vi "G-DataType-To-Go.vi"(8 "error in (no error)":errorcluster, 11 "CMD":variant) -> (0 "error out":errorcluster, 3 "result string":string)   [LabVIEW 2020, in "Generate-Go-CMD.lvlib"]
uses:
  Generate-Go-CMD.lvlib
  <vilib>/Utility/Data Type/NI_Data Type.lvlib
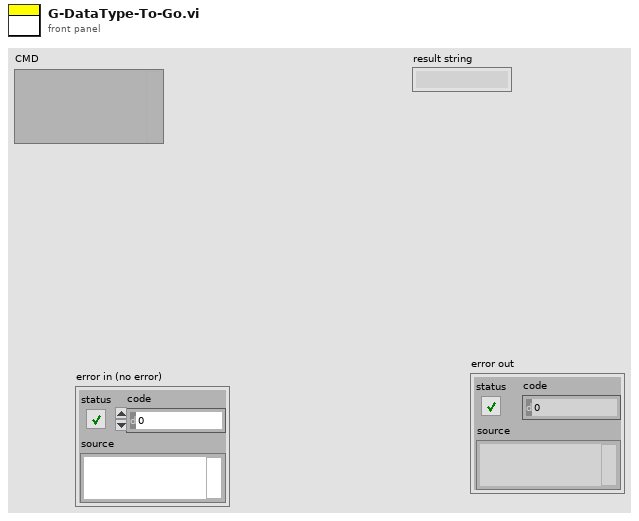
[diagram p1: front panel]
types:
  T1 = typedef "NI_Data Type.lvlib/Data Type.ctl" = enum8{"Invalid Type", "Void", "I8", "I16", "I32", "I64", "U8", "U16", "U32", "U64", "Single Float", "Double Float", "Extended Float", "Single Complex", "Double Complex", "Extended Complex", "Enum U8", "Enum U16", "Enum U32", "Enum U64", "Single Float With Unit", "Double Float With Unit", "Extended Float With Unit", "Single Complex with Unit", "Double Complex with Unit", "Extended Complex with Unit", "Boolean", "String", "Path", "Picture", "Tag", "Array", "Cluster", "Variant", "LV Variant", "Waveform", "Timestamp", "Digital Waveform", "Digital Data", "ExpressData", "Refnum", "External Data", "VI", "Poly VI", "LabVIEW Class Instance", "Fixed Point", "Set Collection", "Map Collection"}
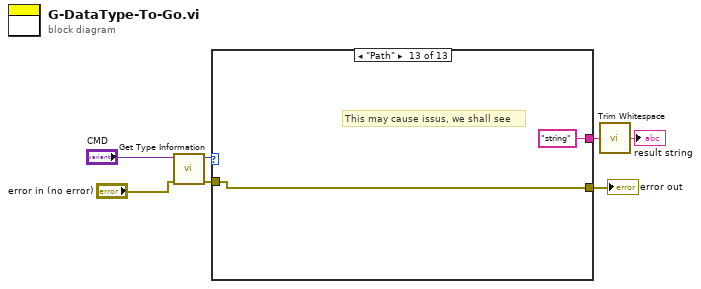
[diagram p0: block diagram]
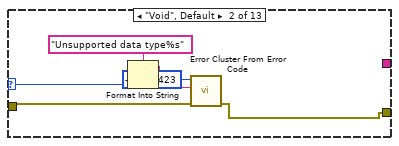
[diagram p3: hidden frame]
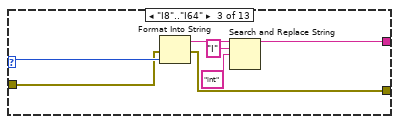
[diagram p4: hidden frame]
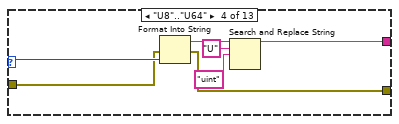
[diagram p5: hidden frame]
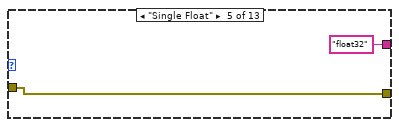
[diagram p6: hidden frame]
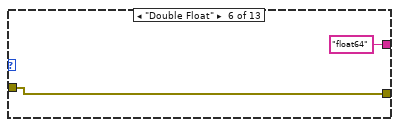
[diagram p7: hidden frame]
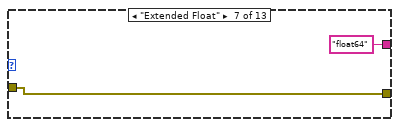
[diagram p8: hidden frame]
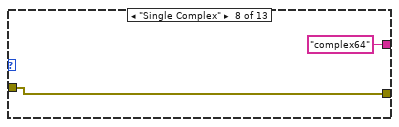
[diagram p9: hidden frame]
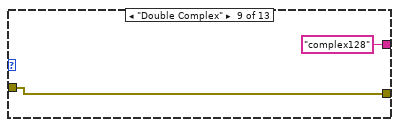
[diagram p10: hidden frame]
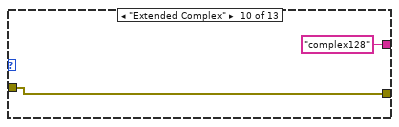
[diagram p11: hidden frame]
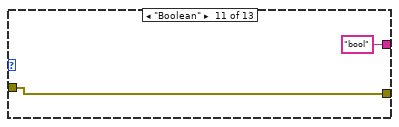
[diagram p12: hidden frame]
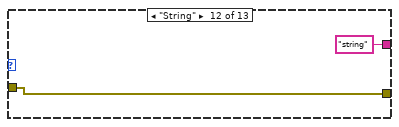
[diagram p13: hidden frame]
diagram:
  n1 = call <vilib>:"Get Type Information.vi"("error in (no error)"="error in (no error)", "variant"="CMD") -> ("error out"=w3:errorcluster, "type"=w5:T1)  [unwired: 5 in, 3 out]
  n2 = case shown="\"Path\"" w5 {
    selector: w5 -> [_ w13 w21 w28 _ _ _ _ _ _ _ _ _]
    tunnel: [_ _ w17 w24 "float32" ("result string") "float64" ("result string") "float64" ("result string") "complex64" ("result string") "complex128" ("result string") "complex128" ("result string") "bool" ("result string") "string" ("result string") "string" ("result string")] -> w4
    tunnel: w3 -> [w8 w14 w16 w23 w29 w31 w33 w35 w37 w39 w41 w43 w45]
    tunnel: [w8 w10 w15 w22 w29 w31 w33 w35 w37 w39 w41 w43 w45] -> w2
    frame "Invalid Type" {
    }
    frame "Void", Default {
      n3 = Format Into String(format string="Unsupported data type%s", w13) -> (resulting string=w12:string)  [unwired: 2 in, 1 out]
      n4 = call <vilib>:"Error Cluster From Error Code.vi"("error in (no error)"=w14, "error message (\"\")"=w12, "error code (0)"=-98328423) -> ("error out"=w10:errorcluster)  [unwired: 6 in]
    }
    frame "I8".."I64" {
      n5 = Format Into String(error in=w16, w21) -> (resulting string=w20:string, error out=w15:errorcluster)  [unwired: 2 in]
      n6 = Search and Replace String(input string=w20, search string="I", replace string="int" ("search string")) -> (result string=w17:string)  [unwired: 5 in, 3 out]
    }
    frame "U8".."U64" {
      n7 = Format Into String(error in=w23, w28) -> (resulting string=w27:string, error out=w22:errorcluster)  [unwired: 2 in]
      n8 = Search and Replace String(input string=w27, search string="U", replace string="uint" ("search string")) -> (result string=w24:string)  [unwired: 5 in, 3 out]
    }
    frame "Single Float" {
    }
    frame "Double Float" {
    }
    frame "Extended Float" {
    }
    frame "Single Complex" {
    }
    frame "Double Complex" {
    }
    frame "Extended Complex" {
    }
    frame "Boolean" {
    }
    frame "String" {
    }
    frame "Path" {
      # "This may cause issus, we shall see"
    }
  }
  "error out" <- w2
  n9 = call <vilib>:"Trim Whitespace.vi"("string"=w4) -> ("trimmed string"=→"result string":string)  [unwired: 1 in]
